vi "Handle.vi"(11 "Base Queue jettl in":refnum<class "Base Queue jettl.lvclass">) -> (2 "Destroy?":bool, 3 "Base Queue jettl out":refnum<class "Base Queue jettl.lvclass">)   [LabVIEW 2021, in "jettl.lvlib" / "Base Queue jettl.lvlib" / "Base Queue jettl.lvclass"]
uses:
  Base Queue jettl.lvclass
  C:/git/jettl/src/jettl/jettl/Queue jettl/Queue jettl.lvclass
  Base Queue jettl.lvclass/Base Queue jettl.ctl
  State/State/State.lvclass
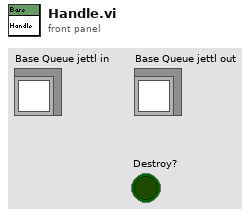
[diagram p1: front panel]
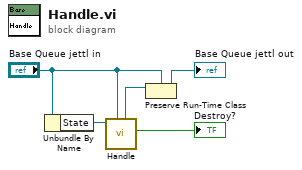
[diagram p0: block diagram]
diagram:
  n1 = Unbundle By Name("Base Queue jettl in") -> ("State"=w5:refnum<class "State.lvclass">)
  n2 = call-dynamic "Handle.vi"("Queue jettl in"="Base Queue jettl in", "State in"=w5) -> ("Destroy?"=→"Destroy?":bool, "Queue jettl out"=w4:refnum<class "Queue jettl.lvclass">)  [unwired: 8 in]
  n3 = Preserve Run-Time Class(object in=w4, 2:"Base Queue jettl in") -> (object out=→"Base Queue jettl out":refnum<class "Base Queue jettl.lvclass">)  [unwired: 1 in, 1 out]
